vi "Unbalanced ANOVA on Rainfall Data.vi"() -> ()   [LabVIEW 2023]
doc: "Uses the 1D ANOVA VI to test the hypothesis that the amount of rainfall does not have an effect on the crop yield for the given experimental data. An ANOVA (analysis of variances) tests the hypothesis that the level of a factor does not have an effect on the experimental outcome. For this example, the amount of rainfall is the factor and is split into 3 levels: 0-L1, L1-L2, and L2-max, where L1 and L2 are controls on the front panel and have units of inches. The experimental outcome is the yield of the crop and has units of bushels."
uses:
  <vilib>/Analysis/NI_AALPro.lvlib
  <vilib>/Analysis/NI_AALBase.lvlib
panel:
  in  "Reject":string="Reject"
  in  "Accept":string="Accept"
  in  "Does not affect the crop":string="The level (amount of rain) does not affect the crop production."
  in  "Affects the crop":string="The level (amount of rain) affects the crop production."
  in  "Tab Control":T1(tab)
  in  "Production (bushels) In":dbl[](array[numeric])=[123.0, 122.0, 126.0, 124.0, 140.0, 141.0, 143.0, 120.0, 118.0, 128.0] format="%#.6g"
  in  "Rain (inches) In":dbl[](array[numeric])=[8.0, 1.0, 1.5, 0.5, 2.5, 3.5, 3.0, 6.0, 8.0, 0.0] format="%#.6g"
  in  "level range control":cluster{dbl, dbl}(slide)={4.0, 2.0} scale=0.0..8.0 scale format="%#.6g"
  out "Number of levels":i32=3
  out "Levels of Rain":i32[](array[numeric])
  out "Rain (inches)":dbl[](array[numeric]) format="%#.6g"
  out "Levels":T2(array[cluster])
  out "Hypothesis of Ho":string
  out "ratio of msa/mse (Fo)":dbl=69.67187500003803 format="%0.4f"
  out "Mean Square Error (MSe)":dbl=5.333333333330562 format="%0.4f"
  out "Sum of Square Factor (SSa)":dbl=743.1666666666861 format="%0.4f"
  out "Mean Square Factor (MSa)":dbl=371.58333333334303 format="%0.4f"
  out "Sum of Squares Error (SSe)":dbl=37.33333333331393 format="%0.4f"
  out "Total Sum of Squares (SSt)":dbl=780.5 format="%#.6g"
  out "Calculated level of significance":dbl=2.3935004415220895e-05 format="%#.6g"
  in  "Level of significance":dbl=0.01
  out "Conclusion:":string
  out "Box Plot":cluster{dbl[], dbl[]}[](graph)
  # "Overview: Demonstrates the use of the 1D ANOVA VI to investigate the effect of rainfall amounts on crop output.\nRequirements: LabVIEW Full Development System\nInstructions:\n1. Verify the parameters on the Problem Statement and Data Entry tabs.\n2. On the Level Classification tab, observe how a continuous measurement is classified in the 3 levels necessary for ANOVA. Also, adjust the level range control to other levels to experiment with different ranges.\n3. Run the VI and analyze the results in the Analysis of Variance and Box Plot tabs."
  # "Statistical analysis:"
  # "Where:\nm : mean value\nt : treatment (or level) effect\ne : measurement error\ni : number of treatments\nj : number of measurements"
  # "Hypothesis:"
  # "Ho : t1 = t2 =t3 =...= ti= 0 against H1 : ti <> 0 for at least one i."
  # "The hypothesis Ho means the measurements are only affected by noise, while the hypothesis H1 means the measurements are affected at least one treatment or level."
  # "Experiment:"
  # "Measure the crop output (in bushels) and the related amount of rain for the specific production."
  # "Preparing the data:"
  # "The amount of rain is a continuous number. To convert to level, we will classify according to the table below:\nlevel 0 (light): min to L1  inches of rain ; level 1 (moderate): L1 to L2 inches of rain ; level 2 (Heavy): L2 to max inches of rain"
  # "(max)"
  # "L2"
  # "L1"
  # "(min)"
  # "Analyzing each level separate:"
  # "After classification, we can evaluate the mean and variance of each level. Notice that the number of measurements for each level is not the same. This kind of experiment is called unbalanced ANOVA."
  # "Analyzing all levels and provide a conclusion :"
  # "Source of\nVariation"
  # "Sum of \nSquares"
  # "Fo"
  # "Mean Square"
  # "Between"
  # "Within"
  # "Total"
  # ">"
  # "?"
  # "Graph the data into a box plot."
  # "Level 0"
  # "Level 1"
  # "Level 2"
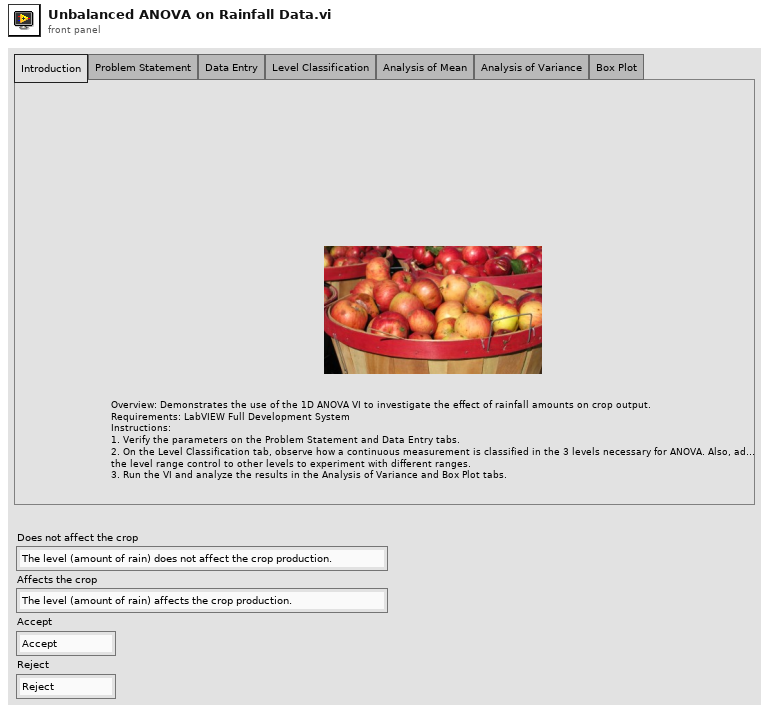
[diagram p1: front panel]
types:
  T1 = enum32{"Introduction", "Problem Statement", "Data Entry", "Level Classification", "Analysis of Mean", "Analysis of Variance", "Box Plot"}
  T2 = cluster{"measurements":dbl[], "total":dbl, "mean":dbl, "variance":dbl}[]
  T3 = cluster{"measurement":dbl[], "mean":dbl, "variance":dbl, "sum":dbl}
  T4 = cluster{"measurement":dbl[], "mean":dbl, "variance":dbl, "sum":dbl}[]
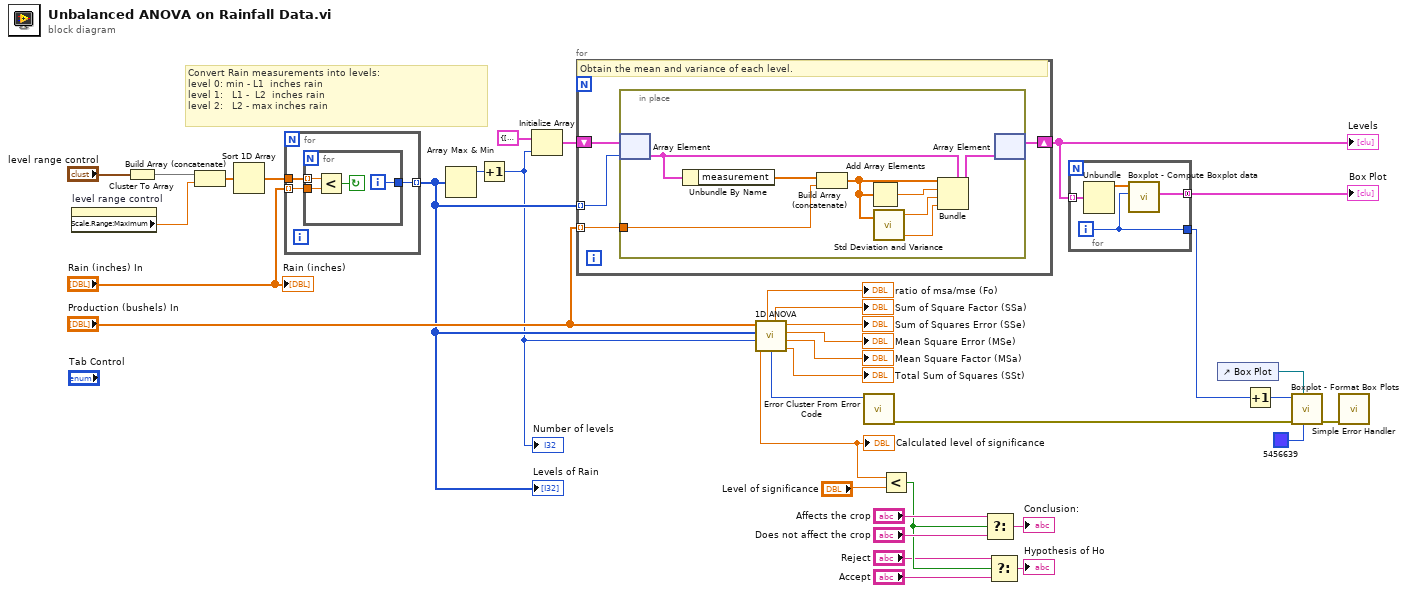
[diagram p0: block diagram]
diagram:
  # "Convert Rain measurements into levels:\nlevel 0: min - L1  inches rain\nlevel 1:   L1 -  L2  inches rain\nlevel 2:   L2 - max inches rain"
  n1 = property on="level range control" class="Slide (strict)"() -> ("Scale.Range:Maximum"=w30:dbl)  [unwired: 2 in, 2 out]
  n2 = Cluster To Array(cluster="level range control") -> (array=w34:dbl[])
  n3 = Build Array (concatenate)(w34, w30) -> (w33:dbl[])
  n4 = Sort 1D Array(array=w33) -> (sorted array=w31:dbl[])
  n5 = for {
    tunnel: w31 -> [w39]
    tunnel: "Rain (inches) In" -> [w38] mode=indexing
    tunnel: [w37] -> w18 mode=indexing
    n6 = for {
      tunnel: w39 -> [w43] mode=indexing
      tunnel: w38 -> [w42]
      tunnel: [w40] -> w37
      i -> [w40]
      stop <- w41 continue-if-true
      n7 = Less?(x=w43, y=w42) -> (x < y?=w41:bool)
    }
  }
  "Levels of Rain" <- w18
  n8 = Array Max & Min(array=w18) -> (max value=w36:i32)  [unwired: 3 out]
  n9 = Increment(x=w36) -> (x+1=w2:i32)
  "Number of levels" <- w2
  n10 = Initialize Array(T3 {"measurement"=[], "mean"=0.0, "variance"=0.0, "sum"=0.0}, w2) -> (w1:T4)
  n11 = for {
    shift-right: [w44] -> w15
    shift-left: w1 -> [w46]
    tunnel: "Production (bushels) In" -> [w47] mode=indexing
    tunnel: w18 -> [w45] mode=indexing
    # "Obtain the mean and variance of each level."
    n12 = in-place {
      in-place-border: w47 -> [w55]
      n13 = in-place-array #1(w46, w45) -> (w49:T3)
      n14 = Unbundle By Name(w49) -> ("measurement"=w54:dbl[])
      n15 = Build Array (concatenate)(w54, w55) -> (w50:dbl[])
      n16 = Add Array Elements(numeric array=w50) -> (sum=w53:dbl)
      n17 = call <vilib>:"Std Deviation and Variance.vi"("X"=w50) -> ("mean"=w52:dbl, "variance"=w51:dbl)  [unwired: 1 in, 1 out]
      n18 = Bundle(cluster=w49, "measurement"=w50, "mean"=w53, "variance"=w52, "sum"=w51) -> (w48:T3)
      n19 = in-place-array #1(w48) -> (w44:T4)  [unwired: 1 out]
    }
  }
  "Levels" <- w15
  n20 = call <vilib>:"1D ANOVA.vi"("# of levels"=w2, "Index"=w18, "X"="Production (bushels) In") -> ("sig A"=w22:dbl, "error"=w29:i32, "tss"=→"Total Sum of Squares (SSt)":dbl, "msa"=→"Mean Square Factor (MSa)":dbl, "f"=→"ratio of msa/mse (Fo)":dbl, "mse"=→"Mean Square Error (MSe)":dbl, "ssa"=→"Sum of Square Factor (SSa)":dbl, "sse"=→"Sum of Squares Error (SSe)":dbl)
  "Calculated level of significance" <- w22
  n21 = call <vilib>:"Error Cluster From Error Code.vi"("error code (0)"=w29) -> ("error out"=w9:errorcluster)  [unwired: 8 in]
  n22 = Less?(x=w22, y="Level of significance") -> (x < y?=w7:bool)
  n23 = Select(t="Affects the crop", s=w7, f="Does not affect the crop") -> (s? t:f=→"Conclusion:":string)
  n24 = Select(t="Reject", s=w7, f="Accept") -> (s? t:f=→"Hypothesis of Ho":string)
  n25 = for {
    tunnel: w15 -> [w59] mode=indexing
    tunnel: [w57] -> w14 mode=concatenating
    tunnel: [w56] -> w13
    i -> [w56]
    n26 = Unbundle(w59) -> ("measurement"=w58:dbl[])  [unwired: 3 out]
    n27 = call "Boxplot - Compute Boxplot data.vi"("Plot number"=w56, "Raw data"=w58) -> ("Boxplot"=w57:cluster{dbl[], dbl[]}[])  [unwired: 9 in]
  }
  "Box Plot" <- w14
  n28 = control-ref of="Box Plot"() -> (w12:refnum<vi>)
  n29 = Increment(x=w13) -> (x+1=w16:i32)
  n30 = call "Boxplot - Format Box Plots.vi"("Plot Color"=u32 5456639 ("Plot.Plot Color"), "XY Graph"=w12, "error in (no error)"=w9, "Number of Plots"=w16) -> ("error out"=w10:errorcluster)  [unwired: 7 in]
  n31 = call <vilib>:"Simple Error Handler.vi"("error in (no error)"=w10) -> ()  [unwired: 4 in, 5 out]
  "Rain (inches)" <- "Rain (inches) In"
